vi "Multistage Multirate Filter Design.vi"() -> ()   [LabVIEW 2023]
doc: "Demonstrates how to use the DFD NStage MRate Filter Design VI to design a multistage multirate filter.\n\nComplete the following steps to use this VI.\n1) Specify the specifications but do not change the <B>Manual Factorization</B> input.\n2) Run the VI.\n3) Change the <B>Frequency Specifications</B> settings, run this VI again, and view the band edge changes.\n4) Change the <B>Ripple Specifications</B> settings, run this VI again, and view the ripple changes in the passband and stopband.\n5) Set different manual factorizations as follows, run the VI, and observe the magnitude response plot for each case.\n a) Remove all values from the <B>Manual Factorization</B> array.\n b) Increase the <B>Manual Factorization</B> array size to 2 and enter values. Ensure that the product of the values equals <B>Factor</B>.\n c) Increase the <B>Manual Factorization</B> array size to 4 and enter values. Ensure that the product of the values equals <B>Factor</B>."
uses:
  <vilib>/addons/Digital Filter Design/_Objects.llb/DFD Multirate Filter Specification (Design).ctl
  <vilib>/addons/Digital Filter Design/_Objects.llb/DFD Filter Ripple Specification (Design).ctl
  <vilib>/addons/Digital Filter Design/_Objects.llb/DFD Multirate Filtering Mode.ctl
  <vilib>/addons/Digital Filter Design/NI_DigFilterLicensed.lvlib
panel:
  out "Error Message":string
  in  "Filtering Mode":T1=2 items=["No Rate Change", "Interpolation", "Decimation"]
  in  "Input Sampling Frequency [Hz]":dbl=64000.0
  in  "Ripple Specifications":T2={"passband"=0.1, "stopband"=60.0, "dB/linear? (T: dB)"=TRUE}
  in  "Frequency Specifications [Hz]":T3={"fpass"=900.0, "fstop"=1100.0}
  in  "Factor":i32=32
  in  "Manual Factorization":i32[](array[numeric])=[2, 4, 4]
  out "Magnitude Responses":cluster{"f0":dbl, "df":dbl, "values":dbl[]}[](graph)
  # "Select Help>>Show Context Help and move the cursor over the VI icon for more information."
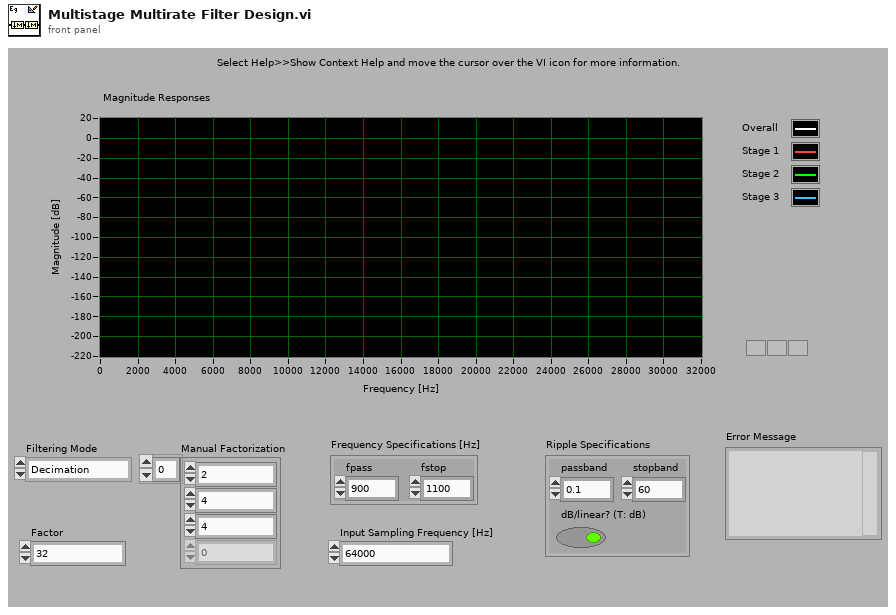
[diagram p1: front panel]
types:
  T1 = typedef "NI_DigFilterLicensed.lvlib/DFD Multirate Filtering Mode.ctl" = u16
  T2 = typedef "NI_DigFilterLicensed.lvlib/DFD Filter Ripple Specification (Design).ctl" = cluster{"passband":dbl, "stopband":dbl, "dB/linear? (T: dB)":bool}
  T3 = typedef "NI_DigFilterLicensed.lvlib/DFD Multirate Filter Specification (Design).ctl" = cluster{"fpass":dbl, "fstop":dbl}
  T4 = typedef "NI_DigFilterLicensed.lvlib/DFD Multirate Filter Obj.ctl" = cluster{"mMRate_Structure":enum16{"CIC", "FIR", "IIR", "Lattice"}, "mMRate_Mode":T5, "mMRate_Factor":i32, "mMRate_FIRParams":cluster{"mMRate_FIR_H":dbl[], "mMRate_FIR_IsNyquist?":bool, "mMRate_FIR_IsSymmetric?":bool}, "mMRate_CICParams":cluster{"mMRate_CIC_#Stage":i32, "mMRate_CIC_Lag":i32, "mMRate_CIC_Type":enum16{"Lowpass", "Highpass"}}, "mMRate_Order":i32, "mMRate_Version":string, "mMRate_Comments":string, "mMRate_RationalFactor":cluster{"mMRate_L":i32, "mMRate_M":i32}, "mMRate_Fs":dbl, "mMRate_Quantized?":bool, "mMRate_QFilterGain":dbl, "mMRate_CoefWl":i16, "mMRate_Scaling":cluster{"mMRate_ScaleByPowerOf2?":bool, "mMRate_ScaleType":T6}, "mMRate_InputWl":i16, "mMRate_OutputWl":i16, "mMRate_OutputMode":T7, "mMRate_MultMode":T8, "mMRate_BitPruning":bool, "mMRate_GainWl":i16, "mMRate_OutputFwl":i16, "mMRate_SumIwl":i16, "mMRate_InputIwl ":i16, "mMRate_SumWl":i16, "mMRate_CoefIwl":i16}
  T5 = typedef "NI_DigFilterLicensed.lvlib/DFD Multirate Mode.ctl" = i16
  T6 = typedef "NI_DigFilterLicensed.lvlib/DFD Coef Norm Type.ctl" = enum16{"No Norm", "Time Domain 1-Norm", "Time Domain 2-Norm", "Time Domain Inf-Norm"}
  T7 = typedef "NI_DigFilterLicensed.lvlib/DFD Round-off Mode.ctl" = enum16{"Nearest", "Truncation"}
  T8 = typedef "NI_DigFilterLicensed.lvlib/DFD FXP MRate Multiply Mode.ctl" = enum16{"Truncated", "Full"}
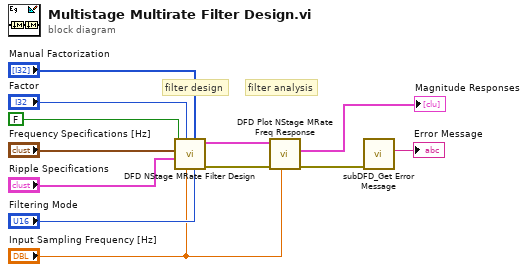
[diagram p0: block diagram]
diagram:
  # "filter analysis"
  # "filter design"
  n1 = call <vilib>:"DFD NStage MRate Filter Design.vi"("filtering mode"="Filtering Mode", "manual factorization"="Manual Factorization", "fs in [Hz]"="Input Sampling Frequency [Hz]", "factor"="Factor", "ripple specs"="Ripple Specifications", "freq specs [Hz]"="Frequency Specifications [Hz]", "using CIC?"=FALSE ("Using CIC?")) -> ("error out"=w11:errorcluster, "multirate filters out"=w12:T4[])  [unwired: 1 in, 2 out]
  n2 = call <vilib>:"DFD Plot NStage MRate Freq Response.vi"("fs in [Hz]"="Input Sampling Frequency [Hz]", "error in (no error)"=w11, "multirate filters in"=w12) -> ("error out"=w1:errorcluster, "magnitude responses"=→"Magnitude Responses":cluster{"f0":dbl, "df":dbl, "values":dbl[]}[])  [unwired: 4 in, 3 out]
  n3 = call <vilib>:"subDFD_Get Error Message.vi"("error in (no error)"=w1) -> ("Error Message"=→"Error Message":string)  [unwired: 10 out]
